vi "Process Thread.vi"(8 "error in (no error)":errorcluster) -> (0 "error out":errorcluster)   [LabVIEW 2020]
doc: "Process thread is used for all internal process"
uses:
  FGV/Controls/FGV_State.ctl
  Controls/Data_Initialize.ctl
  Database/Controls/Account Database.ctl
  Controls/Events_User.ctl
  Database/Controls/Todo.ctl
  SubVIs/Message Queue/Enqueue Message (Single).vi
  <vilib>/Utility/error.llb/Error Cluster From Error Code.vi
  <vilib>/ErrorRing/Error Ring.xnode
  SubVIs/Message Queue/Message Queue.lvlib
types:
  T1 = enum32{"Invalid", "Standard", "Closed", "Hidden", "Minimized", "Maximized"}
  T2 = typedef "FGV_State.ctl" = enum16{"1 - OpenDatabase", "2 - Initialize Events", "3 - Initialize QMH", "4 - Close QMH", "5 - Close Events", "Read FGV", "Save Database", "Def"}
  T3 = typedef "FGV_Data.ctl" = cluster{"QMH":T4, "User Events":T5, "Database":T6[]}
  T4 = typedef "Message Queue.lvlib/All Message Queues.ctl" = cluster{"User Console":refnum<queue>, "Display Console":refnum<queue>, "Sensor Interface":refnum<queue>, "Process":refnum<queue>}
  T5 = typedef "Events_User.ctl" = cluster{"Stop User Console":refnum<user-event>, "Error User Console":refnum<user-event>, "Stop Sensor Interface ":refnum<user-event>, "Error Sensor Interface":refnum<user-event>}
  T6 = typedef "Account Database.ctl" = cluster{"Account Number":i32, "First Name":string, "Last Name":string, "Balance":dbl}
  T7 = typedef "Data_Initialize.ctl" = cluster{"Database":T6[], "User Events":T5}
  T8 = typedef "Todo.ctl" = enum16{"Read", "Update"}
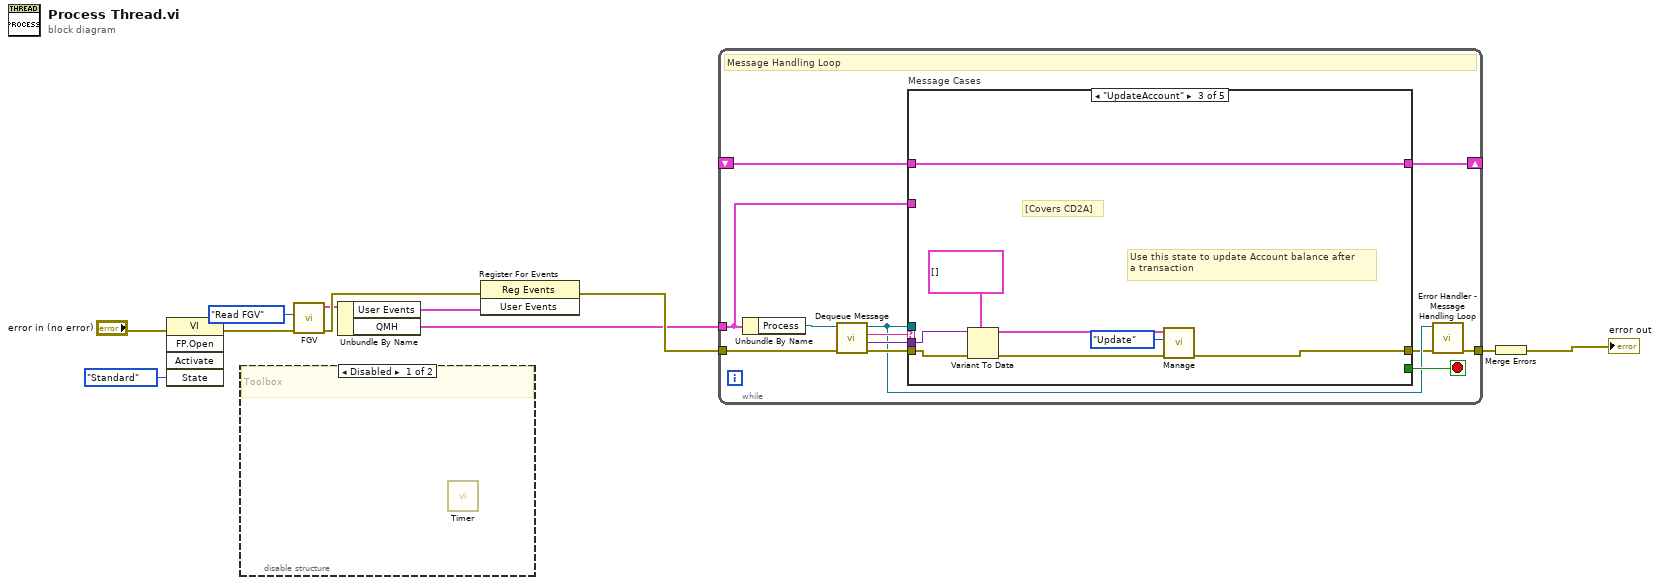
[diagram p0: block diagram]
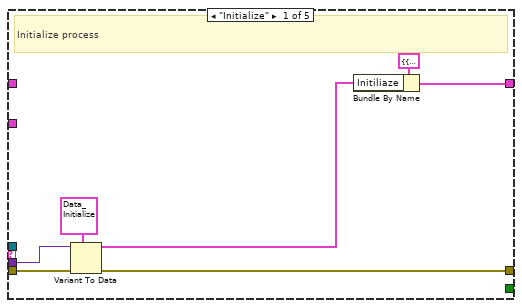
[diagram p3: hidden frame]
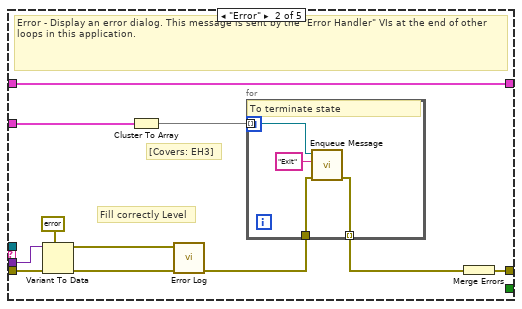
[diagram p4: hidden frame]
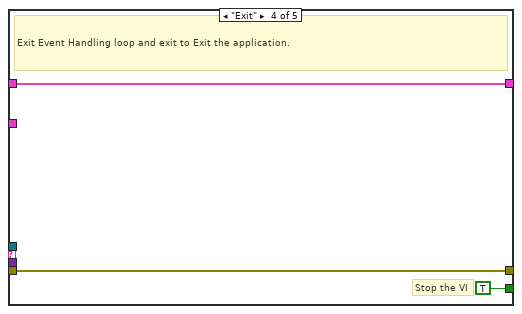
[diagram p5: hidden frame]
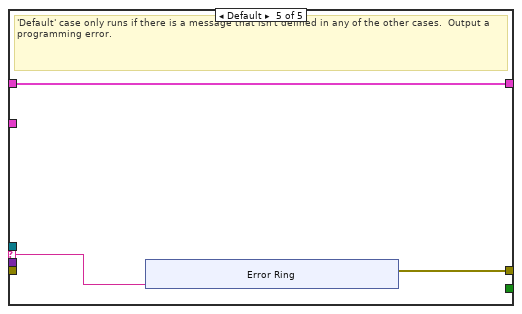
[diagram p6: hidden frame]
diagram:
  n1 = invoke class="VI" method="FP.Open"(error in="error in (no error)", "State"=T1."Standard") -> (error out=w2:errorcluster)  [unwired: 3 in, 4 out]
  n2 = disable-structure shown="Disabled" {
    frame Disabled {
      # "Toolbox"
      n3 = call "Timer.vi"() -> ()  [unwired: 9 in, 3 out]
    }
    frame Enabled {
    }
  }
  n4 = call "FGV.vi"("error in (no error)"=w2, "FGV_State"=FGV_State."Read FGV") -> ("error out"=w8:errorcluster, "FGV 2"=w6:T3)  [unwired: 8 in]
  n5 = Unbundle By Name(w6) -> ("User Events"=w7:T5, "QMH"=w10:T4)
  n6 = register-events(error in=w8, w7) -> (error out=w11:errorcluster)  [unwired: 1 in, 1 out]
  n7 = while {
    tunnel: w10 -> [w12]
    shift-right: [w22] -> _
    shift-left: _ -> [w23]
    tunnel: w11 -> [w20]
    tunnel: [w15] -> w4
    stop <- w21 stop-if-true
    # "Message Handling Loop"
    n8 = Unbundle By Name(w12) -> ("Process"=w13:refnum<queue>)
    n9 = call "Dequeue Message.vi"("error in (no error)"=w20, "Message Queue"=w13) -> ("error out"=w19:errorcluster, "Message Data"=w17:variant, "Message"=w18:string, "dup Message Queue"=w16:refnum<queue>)  [unwired: 6 in]
    n10 = case "Message Cases" shown="\"UpdateAccount\"" w18 {
      selector: w18 -> [_ _ _ _ w57]
      tunnel: w16 -> [_ _ _ _ _]
      tunnel: w19 -> [w28 w41 w52 w54 _]
      tunnel: [w25 w38 w48 w54 w58] -> w14
      tunnel: w23 -> [_ w35 w53 w55 w59]
      tunnel: [w30 w35 w53 w55 w59] -> w22
      tunnel: [_ _ _ TRUE _] -> w21
      tunnel: w17 -> [w24 w40 w51 _ _]
      tunnel: w12 -> [_ w34 _ _ _]
      frame "Initialize" {
        # "Initialize process"
        n11 = Variant To Data(error in=w28, type=T7 {"Database"=[], "User Events"={"Stop User Console"=refnum, "Error User Console"=refnum, "Stop Sensor Interface "=refnum, "Error Sensor Interface"=refnum}} ("Initiliaze"), Variant=w24) -> (data=w26:T7, error out=w25:errorcluster)
        n12 = Bundle By Name(cluster=cluster{"Initiliaze":T7} {"Initiliaze"={"Database"=[], "User Events"={"Stop User Console"=refnum, "Error User Console"=refnum, "Stop Sensor Interface "=refnum, "Error Sensor Interface"=refnum}}} ("Local Data"), "Initiliaze"=w26) -> (w30:cluster{"Initiliaze":T7})
      }
      frame "Error" {
        # "[Covers: EH3]"
        # "Fill correctly Level"
        # "Error - Display an error dialog. This message is sent by the \"Error Handler\" VIs at the end of other loops in this application."
        n13 = Variant To Data(error in=w41, type=errorcluster {"status"=FALSE, "code"=0, "source"=""} ("error constant"), Variant=w40) -> (data=w36:errorcluster, error out=w37:errorcluster)
        n14 = Cluster To Array(cluster=w34) -> (array=w33:refnum<queue>[])
        n15 = call "Error Log.vi"("error in"=w37, "error happened"=w36) -> ("error out"=w32:errorcluster)  [unwired: 9 in]
        n16 = for {
          tunnel: w33 -> [w45] mode=indexing
          tunnel: w32 -> [w44]
          tunnel: [w43] -> w31 mode=indexing
          # "To terminate state"
          n17 = call-poly "Enqueue Message.vi"("error in (no error)"=w44, "Message"="Exit", "Message Queue"=w45) -> ("error out"=w43:errorcluster)  [unwired: 7 in, 1 out]
        }
        n18 = Merge Errors(w31) -> (w38:errorcluster)
      }
      frame "UpdateAccount" {
        # "Use this state to update Account balance after \na transaction"
        # "[Covers CD2A]"
        n19 = Variant To Data(error in=w52, type=T6[] [] ("Database IN"), Variant=w51) -> (data=w47:T6[], error out=w49:errorcluster)
        n20 = call "Manage.vi"("error in"=w49, "ToDo"=Todo."Update", "Database IN"=w47) -> ("error out"=w48:errorcluster)  [unwired: 7 in, 1 out]
      }
      frame "Exit" {
        # "Stop the VI"
        # "Exit Event Handling loop and exit to Exit the application."
      }
      frame Default {
        # "'Default' case only runs if there is a message that isn't defined in any of the other cases.  Output a programming error."
        n21 = xnode "Error Ring"("parameter 0"=w57) -> ("error out"=w58:errorcluster)
      }
    }
    n22 = call "Error Handler - Message Handling Loop.vi"("error in (no error)"=w14, "Message Queue"=w16) -> ("dup error in"=w15:errorcluster)  [unwired: 8 in, 1 out]
  }
  n23 = Merge Errors(w4) -> (→"error out":errorcluster)
